vi "rng+event.vi"() -> ()   [LabVIEW 2022 SP3]
panel:
  in  "[ESC]":bool
  out "Generated Number":dbl
  in  "Generate":bool
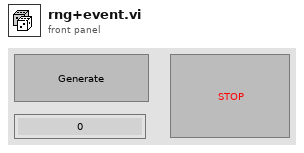
[diagram p1: front panel]
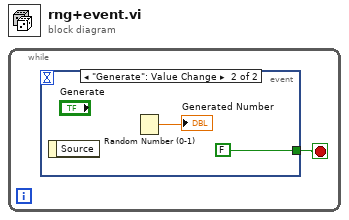
[diagram p0: block diagram]
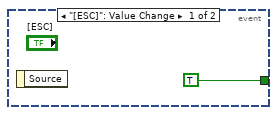
[diagram p2: hidden frame]
diagram:
  n1 = while {
    stop <- w1 stop-if-true
    n2 = event shown="[1] \"Generate\": Value Change" {
      selector: _ -> [_ _]
      dyn-events: _ -> [_ _]
      timeout: _ -> [_ _]
      tunnel: [TRUE FALSE] -> w1
      event "[ESC]": Value Change {
        n3 = event-data() -> ()  [unwired: 1 in, 1 out]
      }
      event "Generate": Value Change {
        n4 = event-data() -> ()  [unwired: 1 in, 1 out]
        n5 = Random Number (0-1)() -> (number: 0 to 1=→"Generated Number":dbl)
      }
    }
  }
